vi "FinalSystem.vi"(8 "error in (no error)":errorcluster, 9 "error in":errorcluster, 10 "FPGA VI Reference Out":refnum<k20>, 11 "Refnum in":refnum<k21>) -> ()   [LabVIEW 2017]
uses:
  <vilib>/rvi/interface/nirviCloseFPGA/nirviCloseFPGA.xnode
  <vilib>/FPGAPlugInAG/Dynamic/niLvFpga_Close_Dynamic.vi
  <vilib>/rvi/interface/nirviReadWriteControl/nirviReadWriteControl.xnode
  NiFpgaLv.dll
  <vilib>/Utility/error.llb/Error Cluster From Error Code.vi
  <vilib>/rvi/interface/Simulation/niFpgaSimulationCallBeginRW.vi
  <vilib>/rvi/errors/niLvFpgaAdjustHostInterfaceError.vi
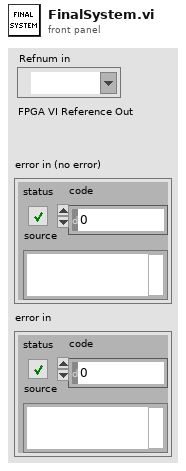
[diagram p1: front panel]
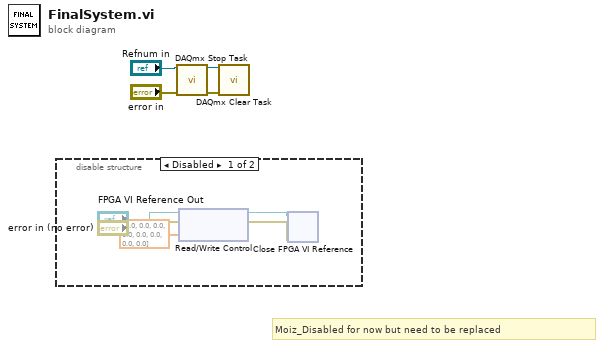
[diagram p0: block diagram]
diagram:
  # "Moiz_Disabled for now but need to be replaced"
  n1 = disable-structure shown="Disabled" {
    frame Disabled {
      n2 = xnode "Read/Write Control"("FPGA VI Reference In"="FPGA VI Reference Out", "error in"="error in (no error)", "AO_Value"=sgl[] [0.0, 0.0, 0.0, 0.0, 0.0, 0.0, 0.0, 0.0]) -> ("FPGA VI Reference Out"=w7:refnum<k20>, "error out"=w8:errorcluster)
      n3 = xnode "Close FPGA VI Reference"("FPGA VI Reference In"=w7, "error in"=w8) -> ()  [unwired: 1 out]
    }
    frame Enabled {
    }
  }
  n4 = call <vilib>:"DAQmx Stop Task.vi"("task/channels in"="Refnum in", "error in"="error in") -> ("task out"=w1:refnum<k21>, "error out"=w4:errorcluster)  [unwired: 12 in]
  n5 = call <vilib>:"DAQmx Clear Task.vi"("task in"=w1, "error in"=w4) -> ()  [unwired: 13 in, 1 out]
